vi "6221+2182等待机柜拷贝.vi"() -> ()   [LabVIEW 2019]
uses:
  <vilib>/Utility/file.llb/Write Delimited Spreadsheet (DBL).vi
  ppms-6621&2182-7001 tunnelling/Keithley 2182/Keithley 2182.lvlib
  ppms-6621&2182-7001 tunnelling/Keithley 622x/Keithley 622x.lvlib
panel:
  in  "2182":refnum<visa-resource-name>
  in  "6221":refnum<visa-resource-name>
  in  "Instrument Type":i32(ring)=3 items=["PPMS", "VersaLab", "DynaCool", "SVSM"]
  out "Measurement Metadata":T1
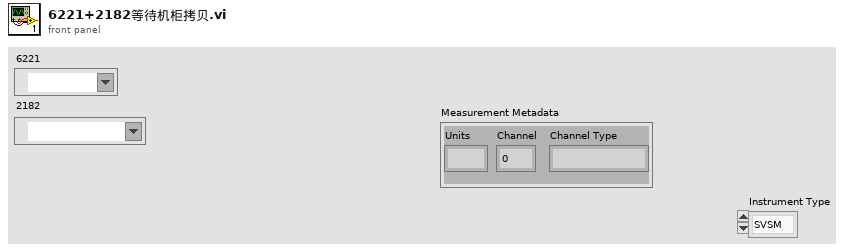
[diagram p1: front panel]
types:
  T1 = cluster{"Units":string, "Channel":i32, "Channel Type":string}
  T2 = enum16{"open", "replace", "create", "open or create", "replace or create", "replace or create with confirmation"}
  T3 = typedef "Keithley 622x.lvlib/KE622x -- Current Level.ctl" = dbl
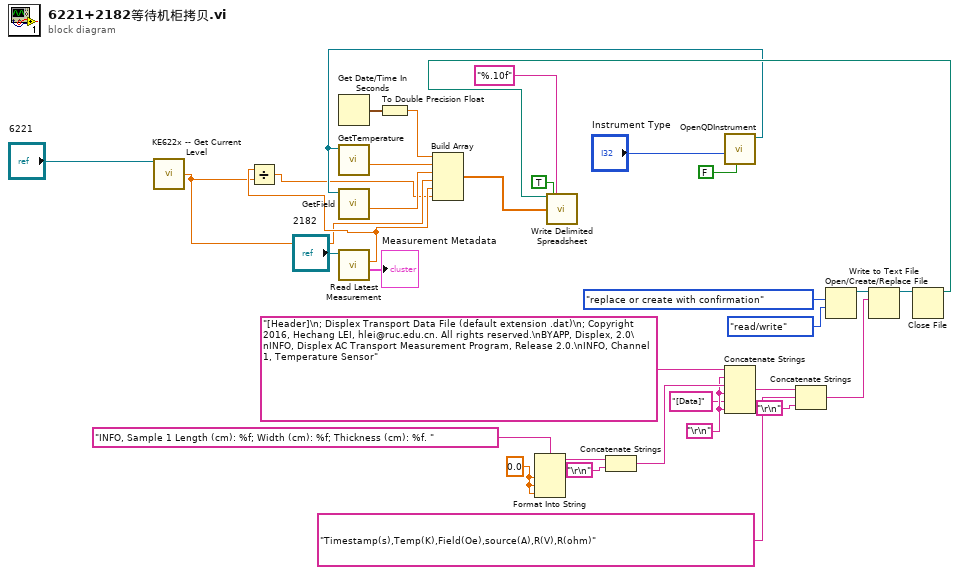
[diagram p0: block diagram]
diagram:
  w21 = 0.0 ("输入 1")
  w18 = "\r\n"
  n1 = call "KE622x -- Get Current Level.vi"("Resource In"="6221") -> ("Current Level (A)"=w2:T3)  [unwired: 12 in, 2 out]
  n2 = Get Date/Time In Seconds() -> (seconds since 1Jan1904=w29:timestamp)
  n3 = call "Read Latest Measurement.vi"("VISA resource name"="2182") -> ("Measurement Metadata"=→"Measurement Metadata":T1, "Measurement"=w3:dbl)  [unwired: 7 in, 2 out]
  n4 = Divide(x=w3, y=w2) -> (x/y=w1:T3)
  n5 = To Double Precision Float(number=w29) -> (double precision float=w28:dbl)
  n6 = Format Into String(format string="INFO, Sample 1 Length (cm): %f; Width (cm): %f; Thickness (cm): %f. " ("string"), w21, w21, w21) -> (resulting string=w23:string)  [unwired: 2 in, 1 out]
  n7 = Concatenate Strings(w23, "\r\n") -> (w25:string)
  n8 = call "OpenQDInstrument.vi"("Remote"=FALSE, "Instrument Type"="Instrument Type") -> ("Instrument Ref"=w6:refnum<k24>)  [unwired: 6 in, 1 out]
  n9 = call "GetTemperature.vi"("Instrument Ref In"=w6) -> ("Temperature"=w33:dbl)  [unwired: 4 in, 4 out]
  n10 = call "GetField.vi"("Instrument Ref In"=w6) -> ("Field"=w32:dbl)  [unwired: 4 in, 4 out]
  n11 = Build Array(w28, w33, w32, w2, w3, w1) -> (w27:T3[])
  n12 = Concatenate Strings("[Header]\n; Displex Transport Data File (default extension .dat)\n; Copyright 2016, Hechang LEI, hlei@ruc.edu.cn. All rights reserved.\nBYAPP, Displex, 2.0\nINFO, Displex AC Transport Measurement Program, Release 2.0.\nINFO, Channel 1, Temperature Sensor" ("string"), w18, w25, w18, "[Data]" ("string"), w18) -> (w24:string)
  n13 = Concatenate Strings(w24, "Timestamp(s),Temp(K),Field(Oe),source(A),R(V),R(ohm)" ("字符串"), "\r\n") -> (w15:string)
  n14 = Open/Create/Replace File(operation (0:open)=T2."replace or create with confirmation" ("操作(0:open)"), access (0:read/write)=enum16{"read/write", "read-only", "write-only"}."read/write" ("权限(0:read/write)")) -> (refnum out=w14:refnum<file>)  [unwired: 4 in, 2 out]
  n15 = Write to Text File(file (use dialog)=w14, text=w15) -> (refnum out=w11:refnum<file>)  [unwired: 2 in, 2 out]
  n16 = Close File(refnum=w11) -> (path=w9:path)  [unwired: 1 in, 1 out]
  n17 = call-poly <vilib>:"Write Delimited Spreadsheet.vi"("file path (dialog if empty)"=w9, "format (%.3f)"="%.10f", "1D data"=w27, "append to file? (new file:F)"=TRUE) -> ()  [unwired: 10 in, 2 out]
